vi "cRIO Benchmarking PC UI.vi"() -> ()   [LabVIEW 2013]
panel:
  out "Double Loopback":dbl
  in  "Color (Yellow(F)/Green(T))":bool
  out "Duration (ns)":dbl(graph)
  out "Output Time":dbl
  out "Process Time":dbl
  out "Input Time":dbl
  in  "Enable LED":bool
  in  "Blinks per Cycle":i32
  in  "Single In":sgl
  in  "Double In":dbl
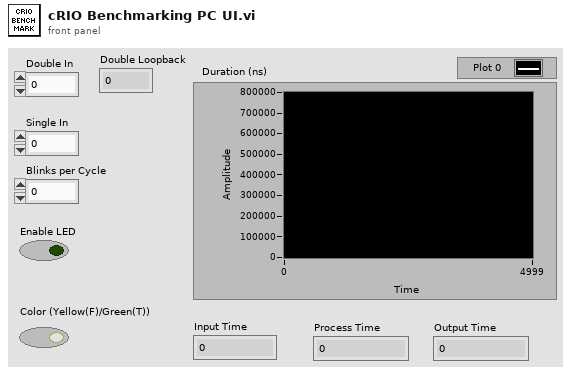
[diagram p1: front panel]
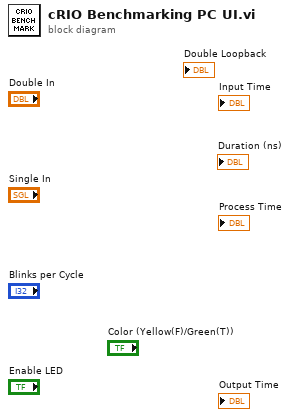
[diagram p0: block diagram]
diagram:
